vi "NI Digital.vi"(8 "error in (no error)":errorcluster, 11 "Message Queues":T3) -> (0 "error out":errorcluster, 3 "Message Queue out":refnum<queue>)   [LabVIEW 2014]
uses:
  support/Message Queue/All Message Queues.ctl
  support/Message Queue/Message Cluster.ctl
  Digital Input Cluster.ctl
  Digital Output Cluster.ctl
  Task.ctl
  <vilib>/DAQmx/read.llb/DAQmx Read (Digital 1D Bool NChan 1Samp 1Line).vi
  <vilib>/DAQmx/write.llb/DAQmx Write (Digital 1D Bool NChan 1Samp 1Line).vi
  support/Message Queue/Lossy Enqueue Message (Single).vi
  <vilib>/DAQmx/miscellaneous.llb/DAQmx Fill In Error Info.vi
  support/Message Queue/Enqueue Message (Single).vi
  <vilib>/Utility/error.llb/Error Cluster From Error Code.vi
  <vilib>/ErrorRing/Error Ring.xnode
  support/Message Queue/Message Queue.lvlib
panel:
  out "Port Write Time [ms]":u32
  out "Port Read Time [ms]":u32
  out "Digital output cluster":T1
  out "Digital input":T2
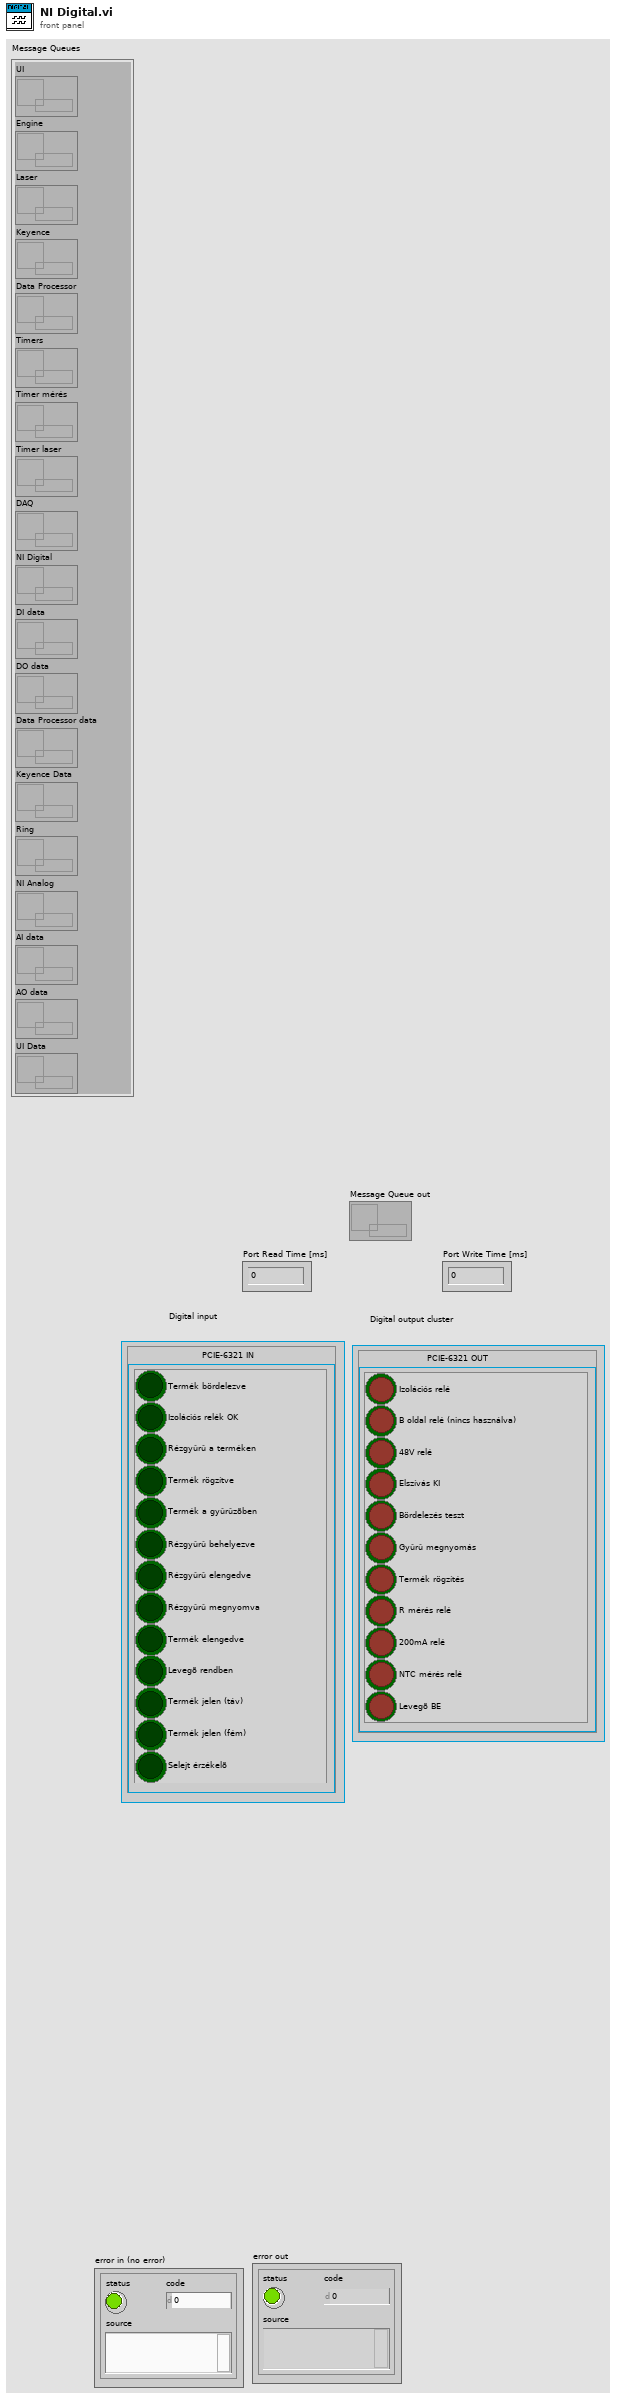
[diagram p1: front panel]
types:
  T1 = typedef "Digital Output Cluster.ctl" = cluster{"PCIE-6321 OUT":cluster{"Izolációs relé":bool, "B oldal relé (nincs használva)":bool, "48V relé":bool, "Elszívás KI":bool, "Bördelezés teszt":bool, "Gyûrû megnyomás":bool, "Termék rögzítés":bool, "R mérés relé":bool, "200mA relé":bool, "NTC mérés relé":bool, "Levegõ BE":bool}}
  T2 = typedef "Digital Input Cluster.ctl" = cluster{"PCIE-6321 IN":cluster{"Termék bördelezve":bool, "Izolációs relék OK":bool, "Rézgyûrû a terméken":bool, "Termék rögzítve":bool, "Termék a gyûrûzõben":bool, "Rézgyûrû behelyezve":bool, "Rézgyûrû elengedve":bool, "Rézgyûrû megnyomva":bool, "Termék elengedve":bool, "Levegõ rendben":bool, "Termék jelen (táv)":bool, "Termék jelen (fém)":bool, "Selejt érzékelõ":bool}}
  T3 = typedef "Message Queue.lvlib/All Message Queues.ctl" = cluster{"UI":refnum<queue>, "Engine":refnum<queue>, "Laser":refnum<queue>, "Keyence":refnum<queue>, "Data Processor":refnum<queue>, "Timers":refnum<queue>, "Timer mérés":refnum<queue>, "Timer laser":refnum<queue>, "DAQ":refnum<queue>, "NI Digital":refnum<queue>, "DI data":refnum<queue>, "DO data":refnum<queue>, "Data Processor data":refnum<queue>, "Keyence Data":refnum<queue>, "Ring":refnum<queue>, "NI Analog":refnum<queue>, "AI data":refnum<queue>, "AO data":refnum<queue>, "UI Data":refnum<queue>}
  T4 = typedef "Task.ctl" = cluster{"Initialized":bool, "task in":refnum<k21>, "task out":refnum<k21>}
  T5 = cluster{"data[0]":bool, "data[1]":bool, "data[2]":bool, "data[3]":bool, "data[4]":bool, "data[5]":bool, "data[6]":bool, "data[7]":bool, "data[8]":bool, "data[9]":bool, "data[10]":bool}
  T6 = cluster{"Izolációs relé":bool, "B oldal relé (nincs használva)":bool, "48V relé":bool, "Elszívás KI":bool, "Bördelezés teszt":bool, "Gyûrû megnyomás":bool, "Termék rögzítés":bool, "R mérés relé":bool, "200mA relé":bool, "NTC mérés relé":bool, "Levegõ BE":bool}
  T7 = cluster{"PCIE-6321 OUT[0]":bool, "PCIE-6321 OUT[1]":bool, "PCIE-6321 OUT[2]":bool, "PCIE-6321 OUT[3]":bool, "PCIE-6321 OUT[4]":bool, "PCIE-6321 OUT[5]":bool, "PCIE-6321 OUT[6]":bool, "PCIE-6321 OUT[7]":bool, "PCIE-6321 OUT[8]":bool, "PCIE-6321 OUT[9]":bool, "PCIE-6321 OUT[10]":bool}
  T8 = cluster{"data[0]":bool, "data[1]":bool, "data[2]":bool, "data[3]":bool, "data[4]":bool, "data[5]":bool, "data[6]":bool, "data[7]":bool, "data[8]":bool, "data[9]":bool, "data[10]":bool, "data[11]":bool, "data[12]":bool}
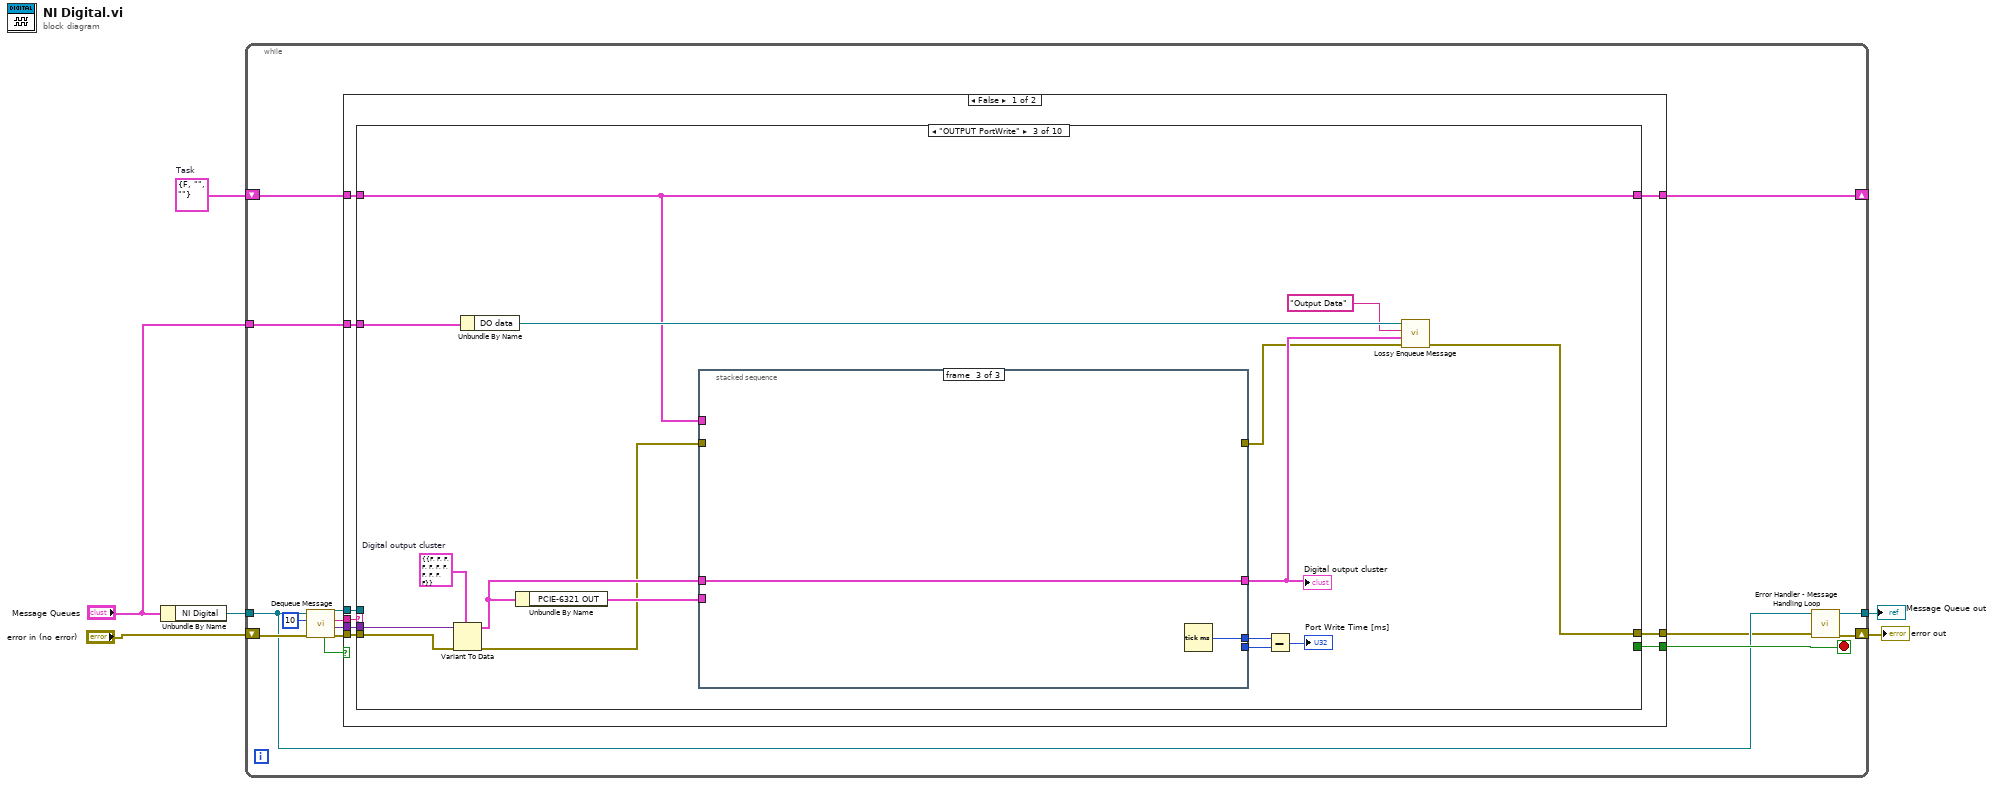
[diagram p0: block diagram]
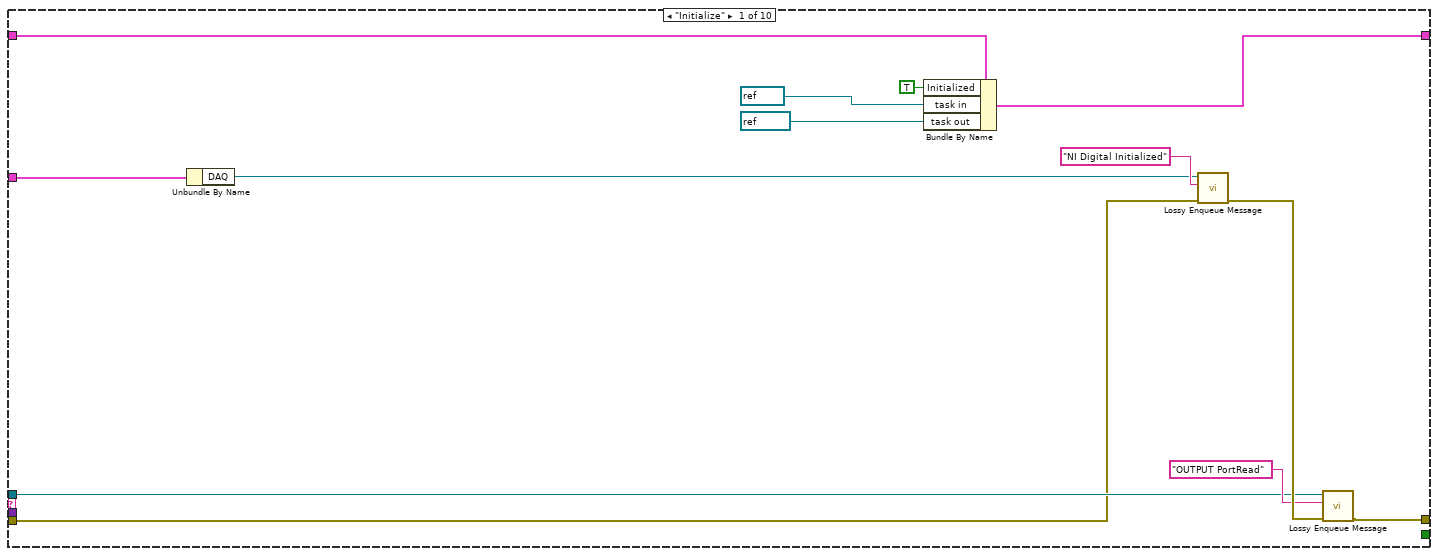
[diagram p2: hidden frame]
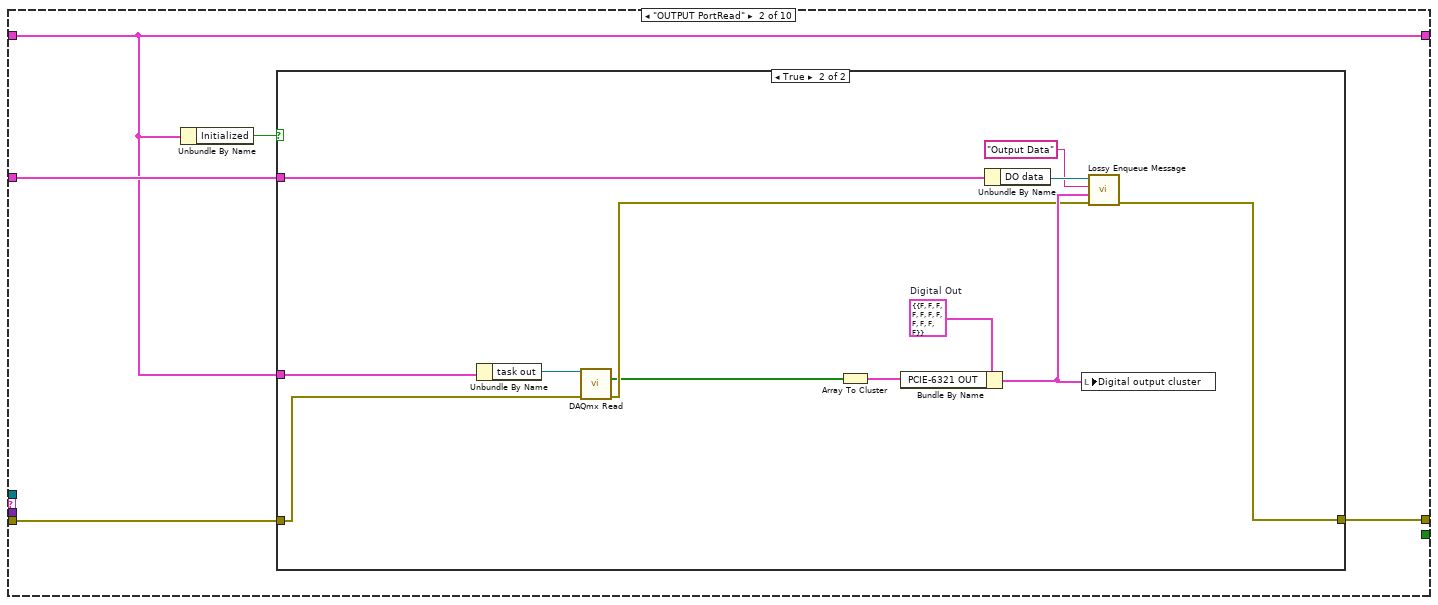
[diagram p3: hidden frame]
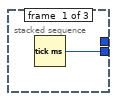
[diagram p5: hidden frame]
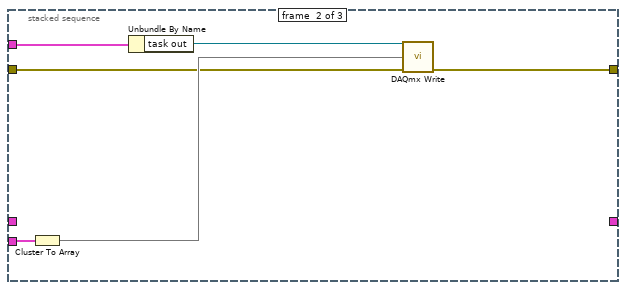
[diagram p6: hidden frame]
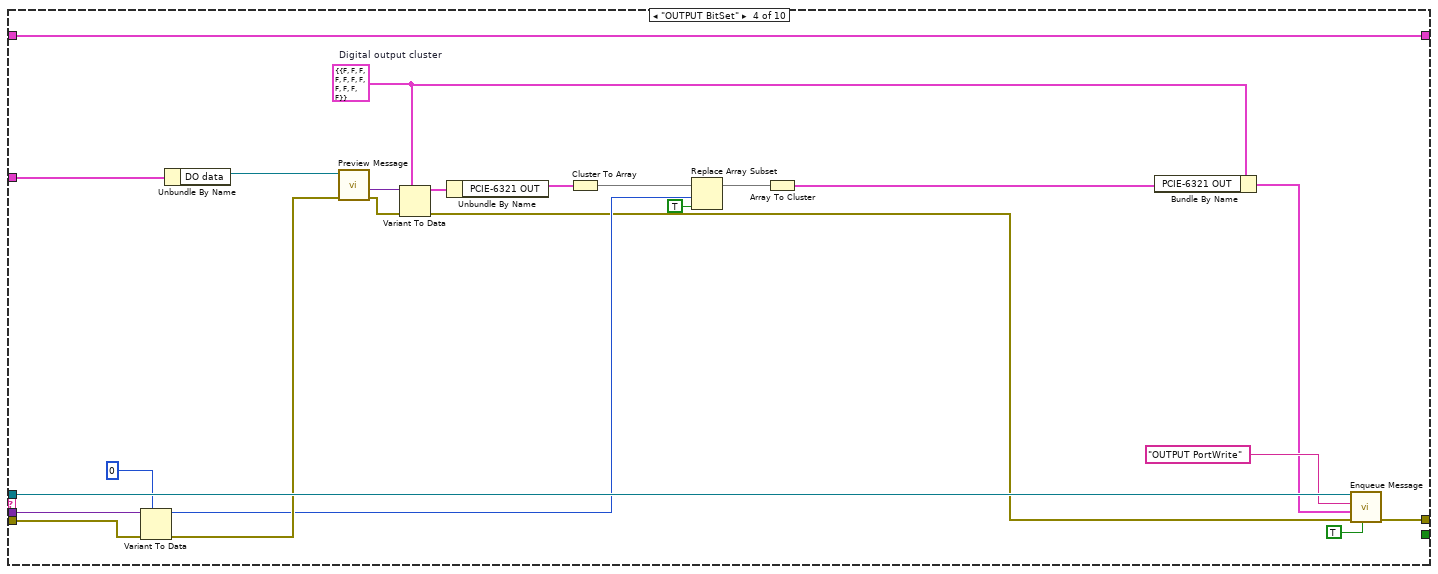
[diagram p7: hidden frame]
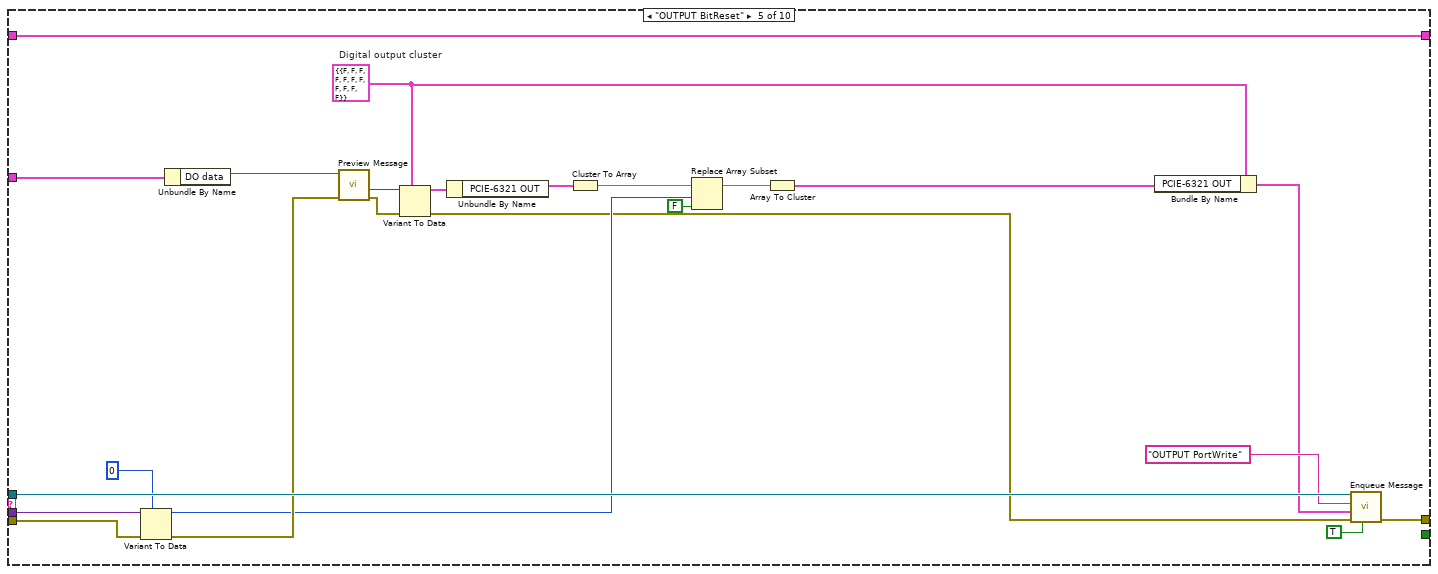
[diagram p8: hidden frame]
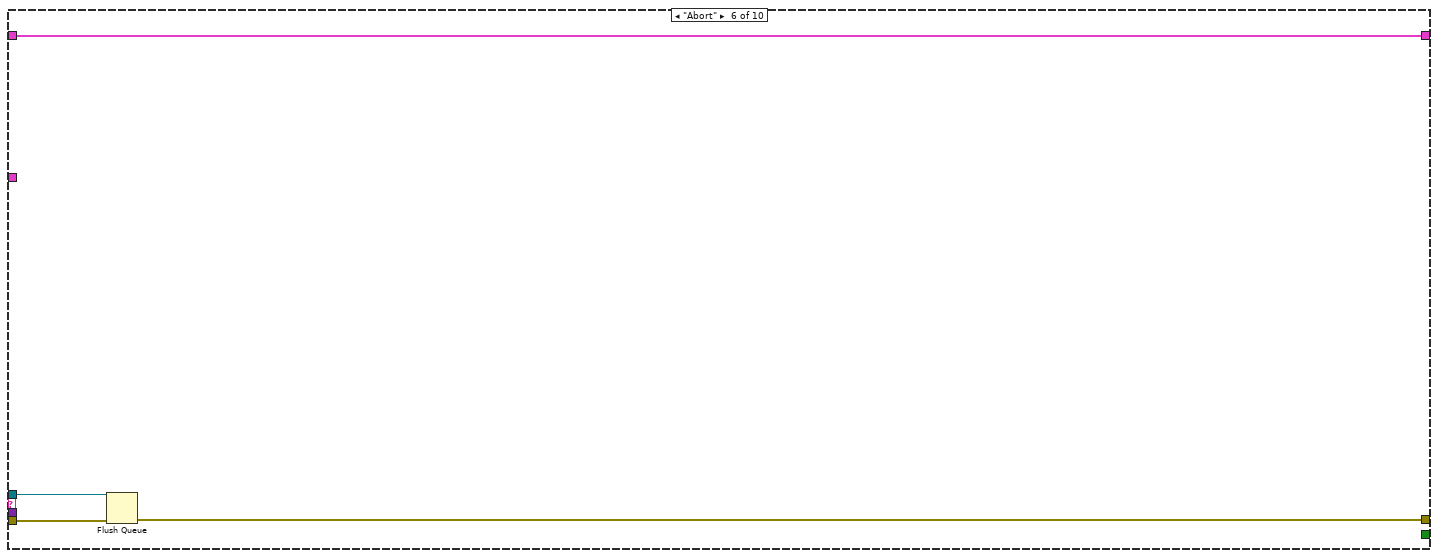
[diagram p9: hidden frame]
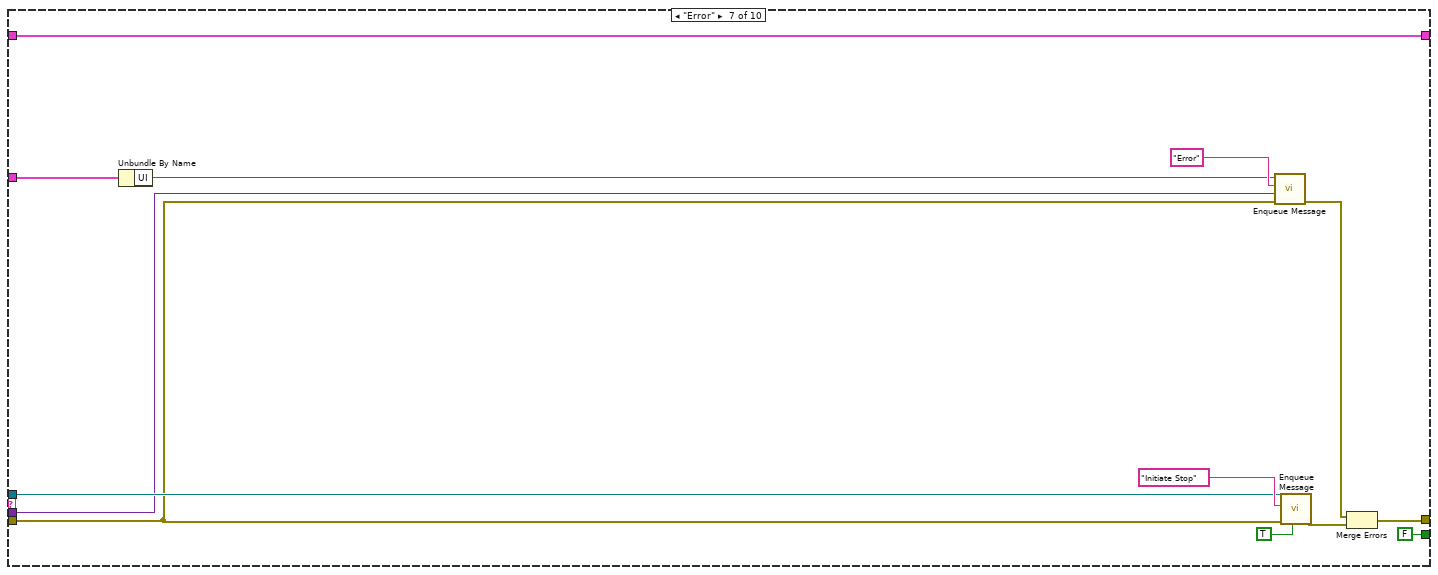
[diagram p10: hidden frame]
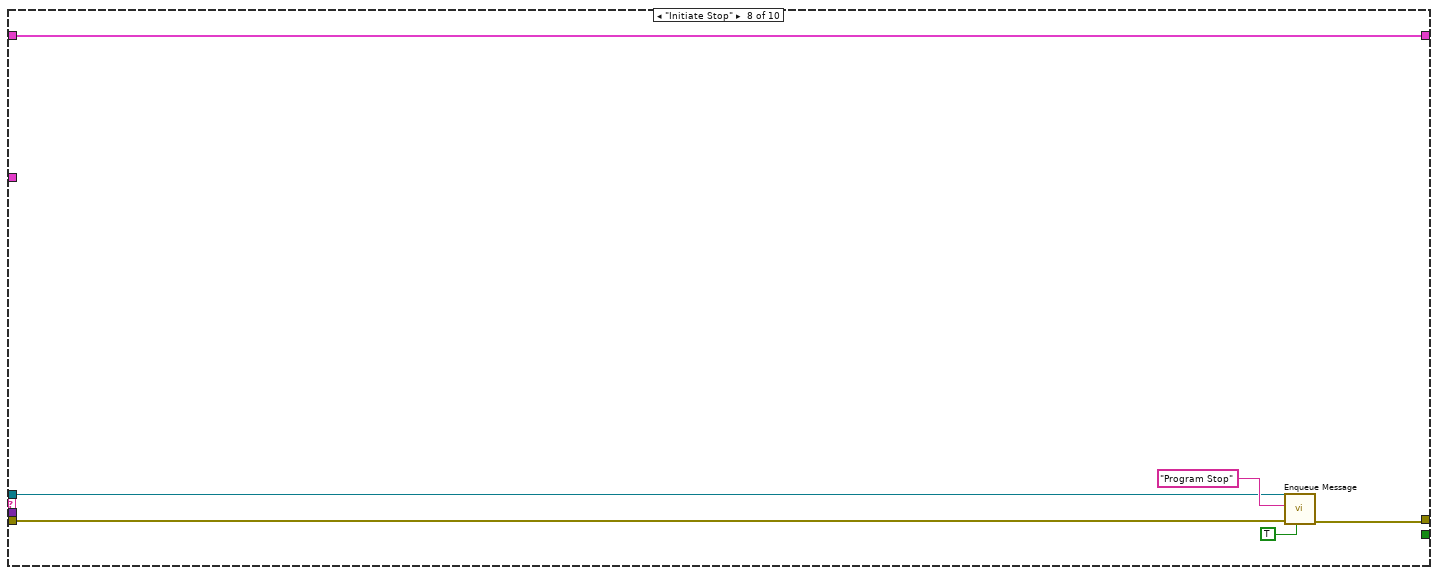
[diagram p11: hidden frame]
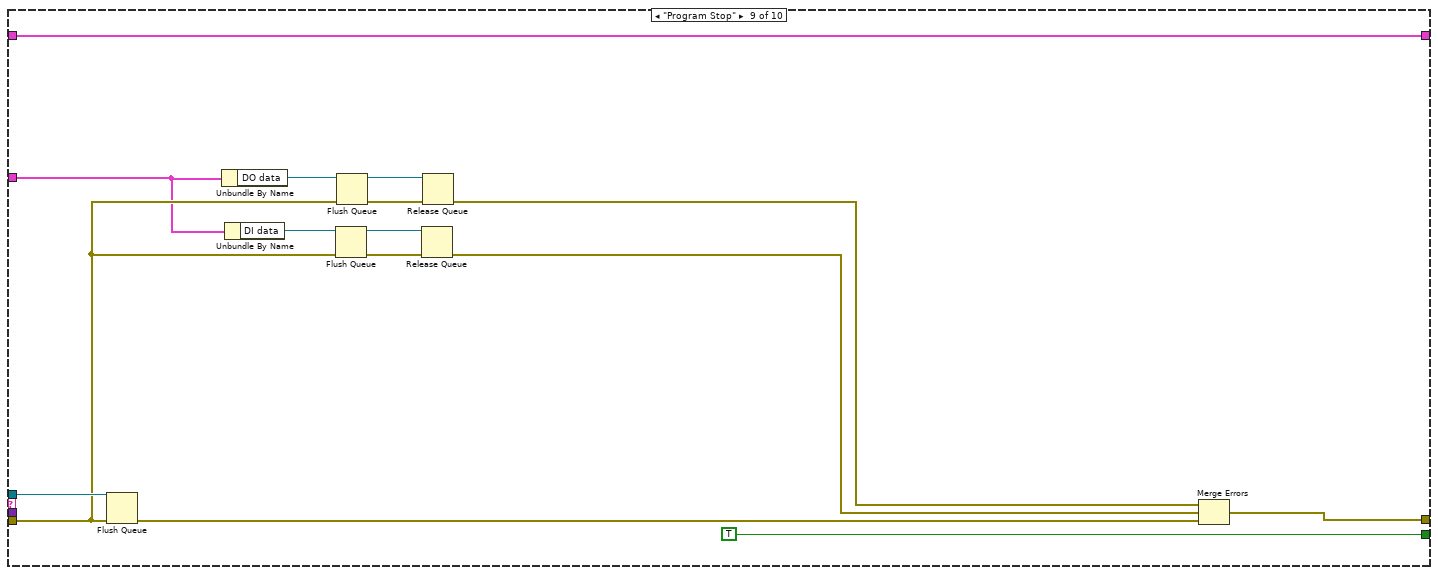
[diagram p12: hidden frame]
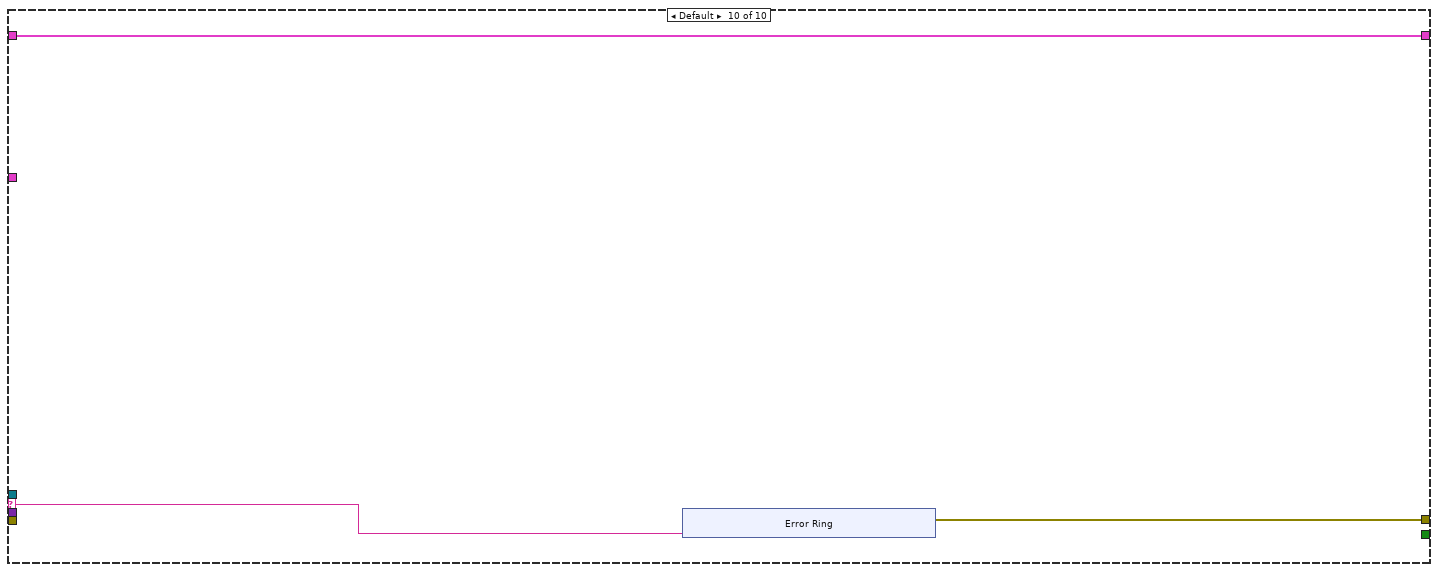
[diagram p13: hidden frame]
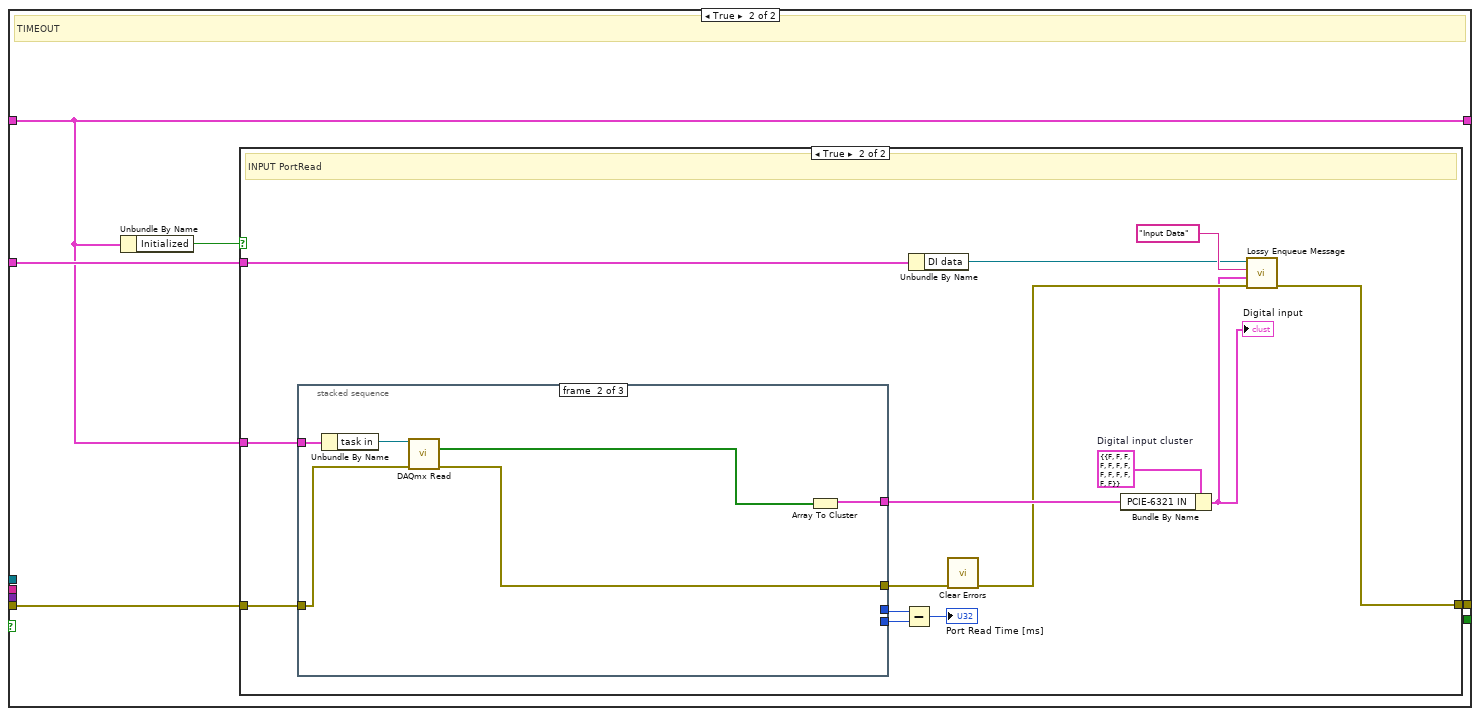
[diagram p14: hidden frame]
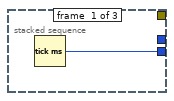
[diagram p16: hidden frame]
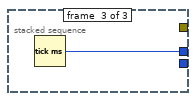
[diagram p17: hidden frame]
diagram:
  w4 = T4 {"Initialized"=FALSE, "task in"="", "task out"=""}  # Task
  n1 = Unbundle By Name("Message Queues") -> ("NI Digital"=w6:refnum<queue>)
  n2 = while {
    tunnel: w6 -> [w12]
    shift-right: [w9] -> _
    shift-left: w4 -> [w8]
    shift-right: [w13] -> w1
    shift-left: "error in (no error)" -> [w21]
    tunnel: "Message Queues" -> [w10]
    tunnel: [w11] -> w5
    stop <- w17 stop-if-true
    n3 = call "Dequeue Message.vi"("error in (no error)"=w21, "timeout in ms (-1)"=10, "Message Queue"=w12) -> ("error out"=w19:errorcluster, "Message Data"=w14:variant, "Message"=w20:string, "dup Message Queue"=w18:refnum<queue>, "timed out?"=w15:bool)  [unwired: 4 in]
    n4 = case shown="False" w15 {
      tunnel: w20 -> [w30 _]
      tunnel: w19 -> [w29 w182]
      tunnel: w18 -> [w28 _]
      tunnel: [w27 _] -> w17
      tunnel: [w26 w184] -> w7
      tunnel: w8 -> [w24 w181]
      tunnel: [w25 w181] -> w9
      tunnel: w14 -> [w23 _]
      tunnel: w10 -> [w22 w185]
      frame False {
        n5 = case shown="\"OUTPUT PortWrite\"" w30 {
          selector: w30 -> [_ _ _ _ _ _ _ _ _ w171]
          tunnel: w29 -> [w32 w48 w76 w107 w130 w134 w139 w150 w161 _]
          tunnel: w28 -> [w36 _ _ w104 w127 w136 w146 w153 w170 _]
          tunnel: [w39 w45 w67 w105 w128 w133 w140 w154 w159 w172] -> w26
          tunnel: [_ _ _ _ _ _ FALSE _ TRUE _] -> w27
          tunnel: [w43 w44 w65 w109 w132 w135 w148 w151 w168 w173] -> w25
          tunnel: w24 -> [w31 w44 w65 w109 w132 w135 w148 w151 w168 w173]
          tunnel: w23 -> [_ _ w77 w108 w131 _ w138 _ _ _]
          tunnel: w22 -> [w42 w46 w75 w106 w129 _ w145 _ w160 _]
          frame "Initialize" {
            n6 = Unbundle By Name(w42) -> ("DAQ"=w40:refnum<queue>)
            n7 = Bundle By Name(cluster=w31, "Initialized"=TRUE, "task in"=refnum<k21> "DI_", "task out"=refnum<k21> "DO_") -> (w43:T4)
            n8 = call-poly "Lossy Enqueue Message.vi"("error in (no error)"=w32, "Message"="NI Digital Initialized", "Message Queue"=w40) -> ("error out"=w38:errorcluster)  [unwired: 7 in, 1 out]
            n9 = call-poly "Lossy Enqueue Message.vi"("error in (no error)"=w38, "Message"="OUTPUT PortRead", "Message Queue"=w36) -> ("error out"=w39:errorcluster)  [unwired: 7 in, 1 out]
          }
          frame "OUTPUT PortRead" {
            n10 = Unbundle By Name(w44) -> ("Initialized"=w47:bool)
            n11 = case shown="True" w47 {
              tunnel: w48 -> [w49 w50]
              tunnel: w46 -> [_ w60]
              tunnel: [w49 w55] -> w45
              tunnel: w44 -> [_ w56]
              frame False {
              }
              frame True {
                w61 = T1 {"PCIE-6321 OUT"={"Izolációs relé"=FALSE, "B oldal relé (nincs használva)"=FALSE, "48V relé"=FALSE, "Elszívás KI"=FALSE, "Bördelezés teszt"=FALSE, "Gyûrû megnyomás"=FALSE, "Termék rögzítés"=FALSE, "R mérés relé"=FALSE, "200mA relé"=FALSE, "NTC mérés relé"=FALSE, "Levegõ BE"=FALSE}}  # Digital Out
                n12 = Unbundle By Name(w56) -> ("task out"=w54:refnum<k21>)
                n13 = call-poly <vilib>:"DAQmx Read.vi"("task/channels in"=w54, "error in"=w50) -> ("data"=w52:bool[], "error out"=w53:errorcluster)  [unwired: 11 in, 1 out]
                n14 = Array To Cluster(array=w52) -> (cluster=w51:T5)
                n15 = Bundle By Name(cluster=w61, "PCIE-6321 OUT"=w51) -> (w57:T1)
                n16 = Unbundle By Name(w60) -> ("DO data"=w59:refnum<queue>)
                n17 = local write "Digital output cluster"(w57) -> ()
                n18 = call-poly "Lossy Enqueue Message.vi"("error in (no error)"=w53, "Message Data"=w57, "Message"="Output Data", "Message Queue"=w59) -> ("error out"=w55:errorcluster)  [unwired: 6 in, 1 out]
              }
            }
          }
          frame "OUTPUT PortWrite" {
            w74 = T1 {"PCIE-6321 OUT"={"Izolációs relé"=FALSE, "B oldal relé (nincs használva)"=FALSE, "48V relé"=FALSE, "Elszívás KI"=FALSE, "Bördelezés teszt"=FALSE, "Gyûrû megnyomás"=FALSE, "Termék rögzítés"=FALSE, "R mérés relé"=FALSE, "200mA relé"=FALSE, "NTC mérés relé"=FALSE, "Levegõ BE"=FALSE}}  # Digital output cluster
            n19 = Variant To Data(error in=w76, type=w74, Variant=w77) -> (data=w64:T1, error out=w63:errorcluster)
            n20 = Unbundle By Name(w75) -> ("DO data"=w73:refnum<queue>)
            n21 = Unbundle By Name(w64) -> ("PCIE-6321 OUT"=w71:T6)
            n22 = stacked-sequence {
              tunnel: w71 -> [_ w83 _]
              tunnel: w63 -> [_ w79 _]
              tunnel: [w78 _ _] -> w69
              tunnel: [_ _ w86] -> w68
              tunnel: w64 -> [_ _ w85]
              tunnel: [_ _ w85] -> w66
              tunnel: w65 -> [_ w84 _]
              tunnel: [_ w80 _] -> w62
              frame #0 {
                n23 = Tick Count (ms)() -> (millisecond timer value=w78:u32)
              }
              frame #1 {
                n24 = Cluster To Array(cluster=w83) -> (array=w82:bool[])
                n25 = Unbundle By Name(w84) -> ("task out"=w81:refnum<k21>)
                n26 = call-poly <vilib>:"DAQmx Write.vi"("task/channels in"=w81, "data"=w82, "error in"=w79) -> ("error out"=w80:errorcluster)  [unwired: 10 in, 2 out]
              }
              frame #2 {
                n27 = Tick Count (ms)() -> (millisecond timer value=w86:u32)
              }
            }
            "Digital output cluster" <- w66
            n28 = Subtract(x=w68, y=w69) -> (x-y=→"Port Write Time [ms]":u32)
            n29 = call-poly "Lossy Enqueue Message.vi"("error in (no error)"=w62, "Message Data"=w66, "Message"="Output Data", "Message Queue"=w73) -> ("error out"=w67:errorcluster)  [unwired: 6 in, 1 out]
          }
          frame "OUTPUT BitSet" {
            w98 = T1 {"PCIE-6321 OUT"={"Izolációs relé"=FALSE, "B oldal relé (nincs használva)"=FALSE, "48V relé"=FALSE, "Elszívás KI"=FALSE, "Bördelezés teszt"=FALSE, "Gyûrû megnyomás"=FALSE, "Termék rögzítés"=FALSE, "R mérés relé"=FALSE, "200mA relé"=FALSE, "NTC mérés relé"=FALSE, "Levegõ BE"=FALSE}}  # Digital output cluster
            n30 = Variant To Data(error in=w107, type=0 ("index of element"), Variant=w108) -> (data=w92:i32, error out=w95:errorcluster)
            n31 = Unbundle By Name(w106) -> ("DO data"=w103:refnum<queue>)
            n32 = call "Preview Message.vi"("error in (no error)"=w95, "Message Queue"=w103) -> ("error out"=w101:errorcluster, "Message Data"=w102:variant)  [unwired: 5 in, 3 out]
            n33 = Variant To Data(error in=w101, type=w98, Variant=w102) -> (data=w99:T1, error out=w90:errorcluster)
            n34 = Unbundle By Name(w99) -> ("PCIE-6321 OUT"=w100:T6)
            n35 = Cluster To Array(cluster=w100) -> (array=w89:bool[])
            n36 = Replace Array Subset(array=w89, new element=TRUE ("new element/subarray"), index=w92) -> (w88:bool[])
            n37 = Array To Cluster(array=w88) -> (cluster=w87:T7)
            n38 = Bundle By Name(cluster=w98, "PCIE-6321 OUT"=w87) -> (w94:T1)
            n39 = call-poly "Enqueue Message.vi"("Priority Message? (F)"=TRUE, "error in (no error)"=w90, "Message Data"=w94, "Message"="OUTPUT PortWrite", "Message Queue"=w104) -> ("error out"=w105:errorcluster)  [unwired: 5 in, 1 out]
          }
          frame "OUTPUT BitReset" {
            w121 = T1 {"PCIE-6321 OUT"={"Izolációs relé"=FALSE, "B oldal relé (nincs használva)"=FALSE, "48V relé"=FALSE, "Elszívás KI"=FALSE, "Bördelezés teszt"=FALSE, "Gyûrû megnyomás"=FALSE, "Termék rögzítés"=FALSE, "R mérés relé"=FALSE, "200mA relé"=FALSE, "NTC mérés relé"=FALSE, "Levegõ BE"=FALSE}}  # Digital output cluster
            n40 = Variant To Data(error in=w130, type=0 ("index of element"), Variant=w131) -> (data=w115:i32, error out=w118:errorcluster)
            n41 = Unbundle By Name(w129) -> ("DO data"=w126:refnum<queue>)
            n42 = call "Preview Message.vi"("error in (no error)"=w118, "Message Queue"=w126) -> ("error out"=w124:errorcluster, "Message Data"=w125:variant)  [unwired: 5 in, 3 out]
            n43 = Variant To Data(error in=w124, type=w121, Variant=w125) -> (data=w122:T1, error out=w113:errorcluster)
            n44 = Unbundle By Name(w122) -> ("PCIE-6321 OUT"=w123:T6)
            n45 = Cluster To Array(cluster=w123) -> (array=w112:bool[])
            n46 = Replace Array Subset(array=w112, new element=FALSE ("new element/subarray"), index=w115) -> (w111:bool[])
            n47 = Array To Cluster(array=w111) -> (cluster=w110:T7)
            n48 = Bundle By Name(cluster=w121, "PCIE-6321 OUT"=w110) -> (w117:T1)
            n49 = call-poly "Enqueue Message.vi"("Priority Message? (F)"=TRUE, "error in (no error)"=w113, "Message Data"=w117, "Message"="OUTPUT PortWrite", "Message Queue"=w127) -> ("error out"=w128:errorcluster)  [unwired: 5 in, 1 out]
          }
          frame "Abort" {
            n50 = Flush Queue(queue=w136, error in (no error)=w134) -> (error out=w133:errorcluster)  [unwired: 2 out]
          }
          frame "Error" {
            n51 = Unbundle By Name(w145) -> ("UI"=w143:refnum<queue>)
            n52 = call-poly "Enqueue Message.vi"("error in (no error)"=w139, "Message Data"=w138, "Message"="Error", "Message Queue"=w143) -> ("error out"=w141:errorcluster)  [unwired: 6 in, 1 out]
            n53 = call-poly "Enqueue Message.vi"("Priority Message? (F)"=TRUE, "error in (no error)"=w139, "Message"="Initiate Stop", "Message Queue"=w146) -> ("error out"=w142:errorcluster)  [unwired: 6 in, 1 out]
            n54 = Merge Errors(w141, w142) -> (w140:errorcluster)
          }
          frame "Initiate Stop" {
            n55 = call-poly "Enqueue Message.vi"("Priority Message? (F)"=TRUE, "error in (no error)"=w150, "Message"="Program Stop", "Message Queue"=w153) -> ("error out"=w154:errorcluster)  [unwired: 6 in, 1 out]
          }
          frame "Program Stop" {
            n56 = Flush Queue(queue=w170, error in (no error)=w161) -> (error out=w158:errorcluster)  [unwired: 2 out]
            n57 = Unbundle By Name(w160) -> ("DO data"=w165:refnum<queue>)
            n58 = Unbundle By Name(w160) -> ("DI data"=w164:refnum<queue>)
            n59 = Flush Queue(queue=w164, error in (no error)=w161) -> (queue out=w163:refnum<queue>, error out=w162:errorcluster)  [unwired: 1 out]
            n60 = Flush Queue(queue=w165, error in (no error)=w161) -> (queue out=w166:refnum<queue>, error out=w167:errorcluster)  [unwired: 1 out]
            n61 = Release Queue(queue=w163, error in (no error)=w162) -> (error out=w157:errorcluster)  [unwired: 1 in, 2 out]
            n62 = Release Queue(queue=w166, error in (no error)=w167) -> (error out=w156:errorcluster)  [unwired: 1 in, 2 out]
            n63 = Merge Errors(w156, w157, w158) -> (w159:errorcluster)
          }
          frame Default {
            n64 = xnode "Error Ring"("parameter 0"=w171) -> ("error out"=w172:errorcluster)
          }
        }
      }
      frame True {
        # "TIMEOUT"
        n65 = Unbundle By Name(w181) -> ("Initialized"=w183:bool)
        n66 = case shown="True" w183 {
          tunnel: w185 -> [_ w189]
          tunnel: w182 -> [w186 w199]
          tunnel: [w186 w196] -> w184
          tunnel: w181 -> [_ w188]
          frame False {
          }
          frame True {
            w200 = T2 {"PCIE-6321 IN"={"Termék bördelezve"=FALSE, "Izolációs relék OK"=FALSE, "Rézgyûrû a terméken"=FALSE, "Termék rögzítve"=FALSE, "Termék a gyûrûzõben"=FALSE, "Rézgyûrû behelyezve"=FALSE, "Rézgyûrû elengedve"=FALSE, "Rézgyûrû megnyomva"=FALSE, "Termék elengedve"=FALSE, "Levegõ rendben"=FALSE, "Termék jelen (táv)"=FALSE, "Termék jelen (fém)"=FALSE, "Selejt érzékelõ"=FALSE}}  # Digital input cluster
            # "INPUT PortRead"
            n67 = stacked-sequence {
              tunnel: w199 -> [_ w203 _]
              tunnel: [_ w207 _] -> w192
              tunnel: [w201 _ _] -> w194
              tunnel: [_ _ w208] -> w195
              tunnel: [_ w202 _] -> w191
              tunnel: w188 -> [_ w206 _]
              frame #0 {
                n68 = Tick Count (ms)() -> (millisecond timer value=w201:u32)
              }
              frame #1 {
                n69 = Unbundle By Name(w206) -> ("task in"=w205:refnum<k21>)
                n70 = call-poly <vilib>:"DAQmx Read.vi"("task/channels in"=w205, "error in"=w203) -> ("data"=w204:bool[], "error out"=w202:errorcluster)  [unwired: 11 in, 1 out]
                n71 = Array To Cluster(array=w204) -> (cluster=w207:T8)
              }
              frame #2 {
                n72 = Tick Count (ms)() -> (millisecond timer value=w208:u32)
              }
            }
            n73 = Subtract(x=w195, y=w194) -> (x-y=→"Port Read Time [ms]":u32)
            n74 = Unbundle By Name(w189) -> ("DI data"=w197:refnum<queue>)
            n75 = call <vilib>:"Clear Errors.vi"("error in (no error)"=w191) -> ("error out"=w190:errorcluster)  [unwired: 5 in, 1 out]
            n76 = Bundle By Name(cluster=w200, "PCIE-6321 IN"=w192) -> (w187:T2)
            "Digital input" <- w187
            n77 = call-poly "Lossy Enqueue Message.vi"("error in (no error)"=w190, "Message Data"=w187, "Message"="Input Data", "Message Queue"=w197) -> ("error out"=w196:errorcluster)  [unwired: 6 in, 1 out]
          }
        }
      }
    }
    n78 = call "Error Handler - Message Handling Loop.vi"("error in (no error)"=w7, "Message Queue"=w12) -> ("dup error in"=w13:errorcluster, "dup Message Queue"=w11:refnum<queue>)  [unwired: 8 in]
  }
  "error out" <- w1
  "Message Queue out" <- w5
